vi "DiffDriveSim_Execute_DiffDrive.vi"(6 "Time":dbl=-1.0, 7 "in DiffDriveTrainSim":T1 {"m_Motor"."Jr_KgM2" format="%13.5p"; "m_Motor"."L_H" format="%13.5p"; "m_Motor"."Kt_NMPerAmp" format="%13.5p"; "m_Motor"."KvINV_RadPerSecPerVolt" format="%13.5p"; "m_Motor"."R_Ohms" format="%13.5p"; "m_Motor"."FreeSpeed_RadPerSec" format="%13.5p"; "m_Motor"."FreeCurrent_Amps" format="%13.5p"; "m_Motor"."StallCurrent_Amps" format="%13.5p"; "m_Motor"."StallTorque_NM" format="%13.5p"; "m_Motor"."nominalVoltage_Volts" format="%13.5p"}, 8 "Actual  Battery Voltage":dbl=12.0, 9 "Nominal Battery Voltage":dbl=12.0, 10 "Right Motor Dmd":dbl, 11 "Left Motor Dmd":dbl) -> (1 "Current Amps":dbl, 2 "Battery Volts":dbl, 3 "out DiffDriveTrainSim":T1 {"m_Motor"."Jr_KgM2" format="%13.5p"; "m_Motor"."L_H" format="%13.5p"; "m_Motor"."Kt_NMPerAmp" format="%13.5p"; "m_Motor"."KvINV_RadPerSecPerVolt" format="%13.5p"; "m_Motor"."R_Ohms" format="%13.5p"; "m_Motor"."FreeSpeed_RadPerSec" format="%13.5p"; "m_Motor"."FreeCurrent_Amps" format="%13.5p"; "m_Motor"."StallCurrent_Amps" format="%13.5p"; "m_Motor"."StallTorque_NM" format="%13.5p"; "m_Motor"."nominalVoltage_Volts" format="%13.5p"})   [LabVIEW 2019]
uses:
  <vilib>/Rock Robotics/WPI/ThirdParty/JAS_Junk/TrajLib/TypeDef/DIFF_DRIVE_TRAIN_SIM.ctl
  <vilib>/Rock Robotics/WPI/ThirdParty/JAS_Junk/TrajLib/TypeDef/LINEAR_SYSTEM.ctl
  <vilib>/Analysis/Matrix/Datatypes/RealMatrix.ctl
  <vilib>/Rock Robotics/WPI/ThirdParty/JAS_Junk/TrajLib/TypeDef/DCMOTOR.CTL
  <vilib>/Rock Robotics/WPI/ThirdParty/JAS_Junk/TrajLib/Trajectory_Library.lvlib
  Simulated_Field/Simulated_Field.lvlib
  <vilib>/Analysis/Matrix/NI_Matrix.lvlib
panel:
  # "<States, 1>"
  # "<Outputs, 1>"
  # "<Inputs, 1>"
  # "<Outputs, 1>"
  # "<States,States>"
  # "<States,Inputs>"
  # "<Outputs,States>"
  # "<Outputs,Inputs>"
  # "<States, 1>"
  # "<Outputs, 1>"
  # "<Inputs, 1>"
  # "<Outputs, 1>"
  # "<States,States>"
  # "<States,Inputs>"
  # "<Outputs,States>"
  # "<Outputs,Inputs>"
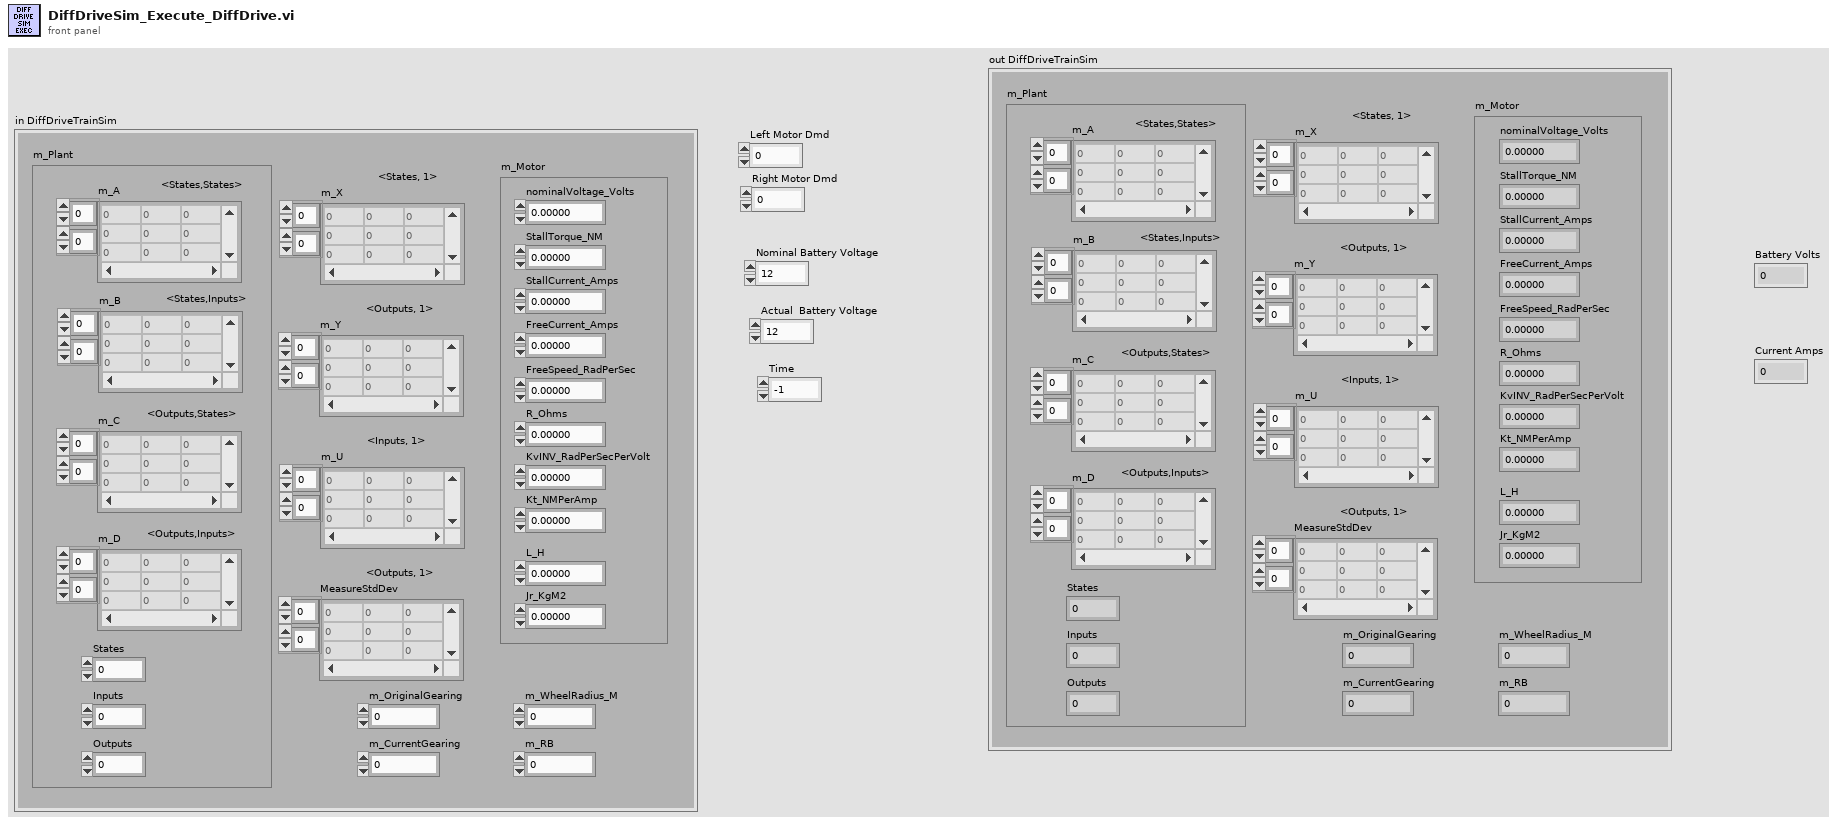
[diagram p1: front panel]
types:
  T1 = typedef "Trajectory_Library.lvlib/DIFF_DRIVE_TRAIN_SIM.ctl" = cluster{"m_Plant":T2, "m_X":T3, "m_Y":T3, "m_U":T3, "MeasureStdDev":T3, "m_Motor":T4, "m_OriginalGearing":dbl, "m_CurrentGearing":dbl, "m_WheelRadius_M":dbl, "m_RB":dbl}
  T2 = typedef "Trajectory_Library.lvlib/LINEAR_SYSTEM.ctl" = cluster{"m_A":T3, "m_B":T3, "m_C":T3, "m_D":T3, "States":i32, "Inputs":i32, "Outputs":i32}
  T3 = typedef "NI_Matrix.lvlib/RealMatrix.ctl" = dbl[][]
  T4 = typedef "Trajectory_Library.lvlib/DCMOTOR.CTL" = cluster{"nominalVoltage_Volts":dbl, "StallTorque_NM":dbl, "StallCurrent_Amps":dbl, "FreeCurrent_Amps":dbl, "FreeSpeed_RadPerSec":dbl, "R_Ohms":dbl, "KvINV_RadPerSecPerVolt":dbl, "Kt_NMPerAmp":dbl, "L_H":dbl, "Jr_KgM2":dbl}
  T5 = typedef "Trajectory_Library.lvlib/POSE2D.ctl" = cluster{"TRANSLATION":T6, "ROTATION":T7}
  T6 = typedef "Trajectory_Library.lvlib/TRANSLATION2D.ctl" = cluster{"X":dbl, "Y":dbl}
  T7 = typedef "Trajectory_Library.lvlib/ROTATION2D.ctl" = cluster{"VALUE":dbl, "COS":dbl, "SIN":dbl}
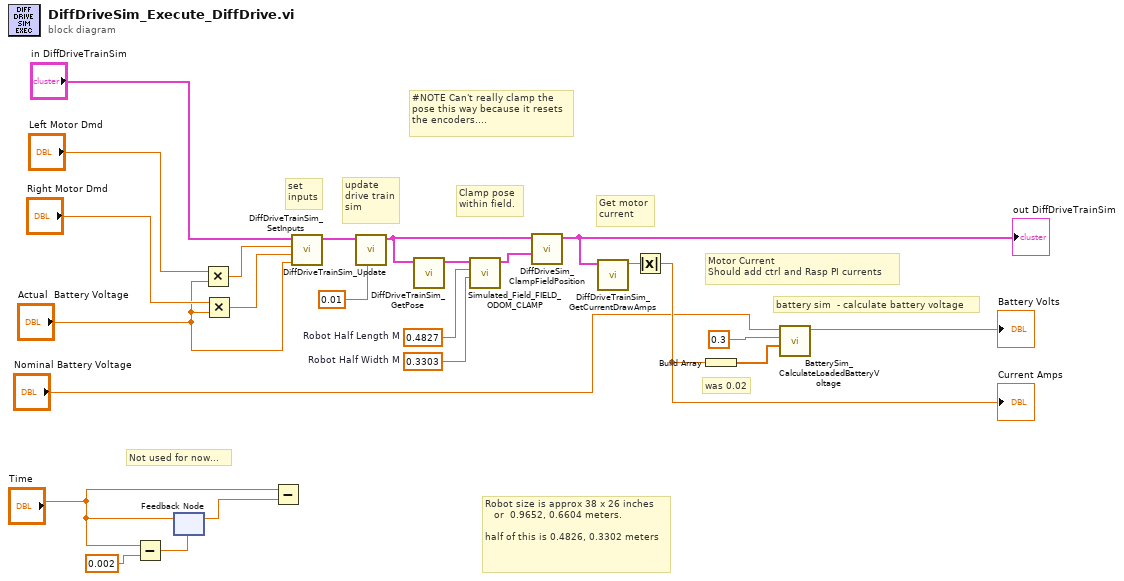
[diagram p0: block diagram]
diagram:
  w4 = 0.4827  # Robot Half Length M
  w5 = 0.3303  # Robot Half Width M
  # "#NOTE Can't really clamp the \npose this way because it resets\nthe encoders...."
  # "Robot size is approx 38 x 26 inches\n   or  0.9652, 0.6604 meters.\n\nhalf of this is 0.4826, 0.3302 meters"
  # "Not used for now..."
  # "Clamp pose\nwithin field."
  # "was 0.02"
  # "Get motor\ncurrent"
  # "Motor Current\nShould add ctrl and Rasp PI currents"
  # "update\ndrive train\nsim"
  # "set\ninputs"
  # "battery sim  - calculate battery voltage"
  n1 = Subtract(x="Time", y=0.002) -> (x-y=w9:dbl)
  n2 = feedback-in #1("Time") -> ()
  n3 = feedback #1(w9) -> (w8:dbl)
  n4 = Multiply(x="Left Motor Dmd", y="Actual  Battery Voltage") -> (x*y=w21:dbl)
  n5 = Multiply(x="Right Motor Dmd", y="Actual  Battery Voltage") -> (x*y=w22:dbl)
  n6 = Subtract(x="Time", y=w8) -> ()  [unwired: 1 out]
  n7 = call <vilib>:"DiffDriveTrainSim_SetInputs.vi"("BatteryVoltage"="Actual  Battery Voltage", "Right_Volts"=w22, "Left_Volts"=w21, "in DiffDriveTrainSim"="in DiffDriveTrainSim") -> ("out DiffDriveTrainSim"=w16:T1)  [unwired: 6 in, 1 out]
  n8 = call <vilib>:"DiffDriveTrainSim_Update.vi"("dT_Seconds"=0.01, "in DiffDriveTrainSim"=w16) -> ("out DiffDriveTrainSim"=w3:T1)  [unwired: 8 in, 1 out]
  n9 = call <vilib>:"DiffDriveTrainSim_GetPose.vi"("DiffDriveTrainSim"=w3) -> ("Pose"=w6:T5)  [unwired: 10 in]
  n10 = call "Simulated_Field_FIELD_ODOM_CLAMP.vi"("Robot Half Width M"=w5, "Robot Half Length M"=w4, "in Sim Pose"=w6) -> ("out Sim Pose"=w1:T5)  [unwired: 8 in]
  n11 = call "DiffDriveSim_ClampFieldPosition.vi"("new Sim Pose"=w1, "in DiffDriveTrainSim"=w3) -> ("out DiffDriveTrainSim"=w2:T1)  [unwired: 9 in]
  "out DiffDriveTrainSim" <- w2
  n12 = call <vilib>:"DiffDriveTrainSim_GetCurrentDrawAmps.vi"("DiffDriveTrainSim"=w2) -> ("TotalCurrent_Amps"=w19:dbl)  [unwired: 10 in]
  n13 = Absolute Value(x=w19) -> (abs(x)=w20:dbl)
  "Current Amps" <- w20
  n14 = Build Array(w20) -> (w18:dbl[])
  n15 = call <vilib>:"BatterySim_CalculateLoadedBatteryVoltage.vi"("Currents"=w18, "Resistance_Ohms"=0.3, "NominalVoltage"="Nominal Battery Voltage") -> ("Voltage"=→"Battery Volts":dbl)  [unwired: 8 in]
